vi "StateShooter.vi"(0 "Master State In":T1(ring)) -> ()   [LabVIEW 2023]
doc: "This VI performs all of the calculations and decisions related to the swerve drive."
uses:
  <vilib>/Rock Robotics/WPI/DriverStation/WPI_DriverStationAllianceInfo.ctl
  52ab7f25-ced8-4b52-a2db-c1468d392cc7.vi
  GlobalDriverStationCommands.vi
  GlobalShooter.vi
  GlobalNoteHandling.vi
  GlobalPoseAndTargeting.vi
  GlobalDriverStationData.vi
  GlobalAutonomous.vi
  GlobalElevator.vi
panel:
  in  "Stage Shooter Command":dbl=0.35 format="%#_13g"
  in  "StageAngle":dbl
  in  "AMP Shooter Command":dbl=0.5 format="%#_13g"
  in  "Speaker Height":dbl=65.0 format="%#_13g"
  in  "Shooter Ratio":dbl=-0.576 format="%#_13g"
  in  "Shooter Command":dbl=0.7 format="%#_13g"
  in  "Wrist Default angle (deg)":dbl=27.0 format="%#_13g"
  in  "Shooter Firing Duration (ms)":u32=500
  in  "Trap Wrist Angle":dbl
  in  "Climbing Wrist Angle":dbl=54.0
  in  "Amp Wrist Angle":dbl=72.0
  in  "Acceptable Wrist Error (deg)":dbl=2.0
  in  "Maximum Shooter Range (in)":dbl=240.0
  in  "Acceptable Heading Error (deg)":dbl=5.0 format="%#_13g"
  in  "Shooter_Acceptable_Velocity_Speaker (RPM)":dbl=1000.0
  in  "Prespin Duration (ms)":u32=2000
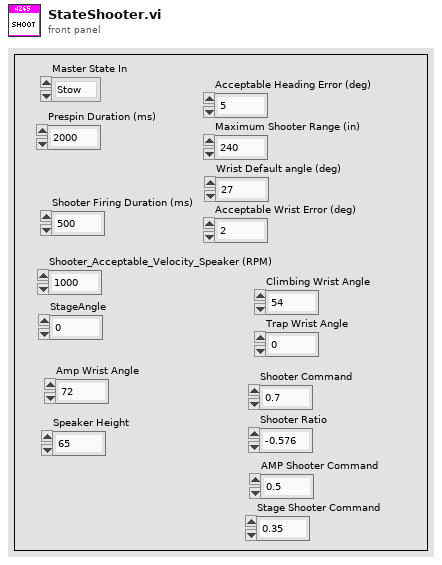
[diagram p1: front panel]
types:
  T1 = enum16{"Stow", "Speaker", "Amp", "Climbing", "Trap"}
  T2 = typedef "WPI_DriverStationAllianceInfo.ctl" = enum16{"Red", "Blue", "Invalid"}
  T3 = enum16{"Safety", "Travelling", "Positioning", "Holding"}
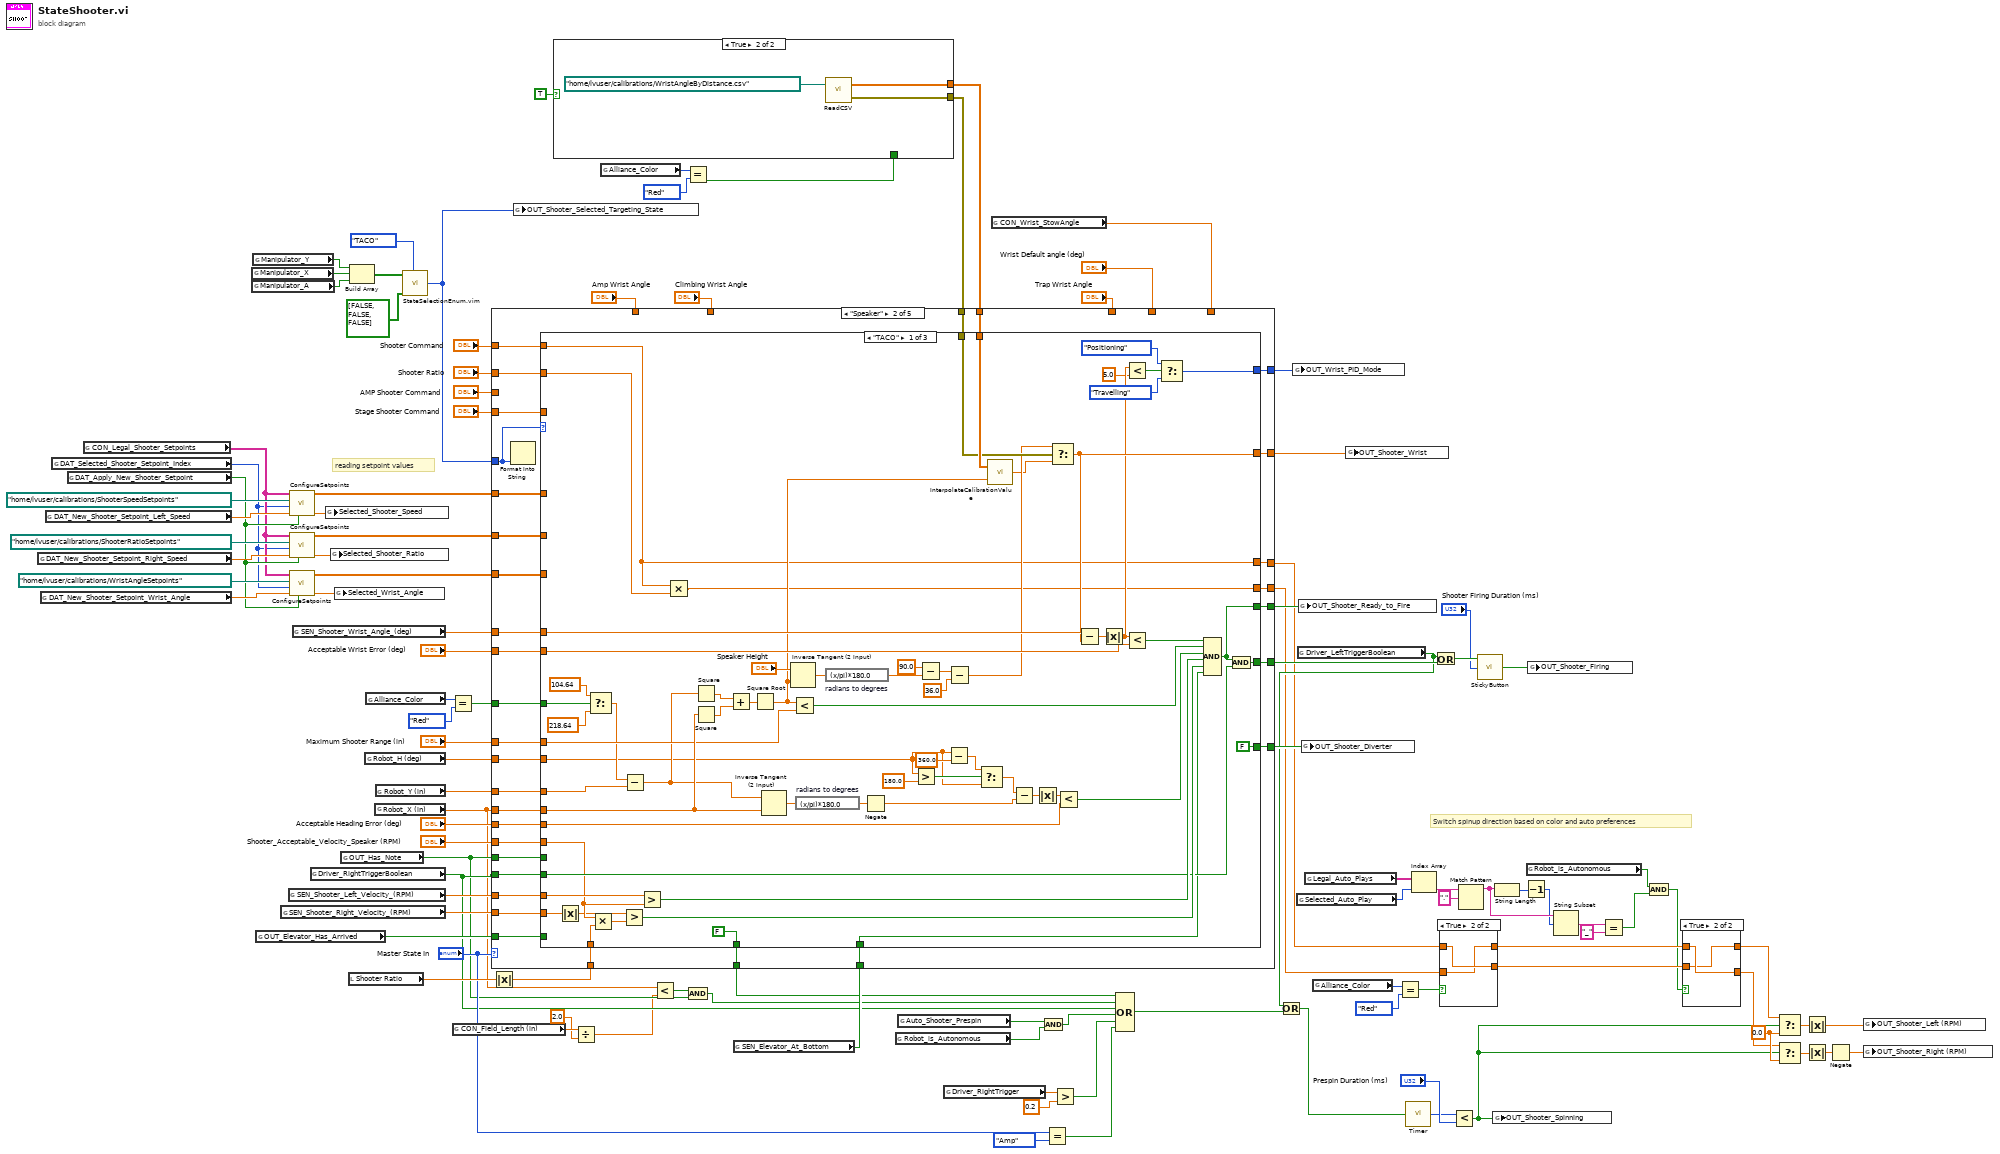
[diagram p0: block diagram]
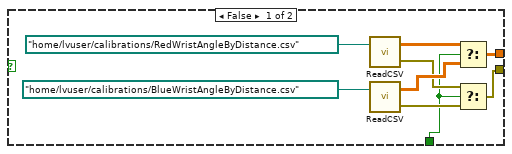
[diagram p4: hidden frame]
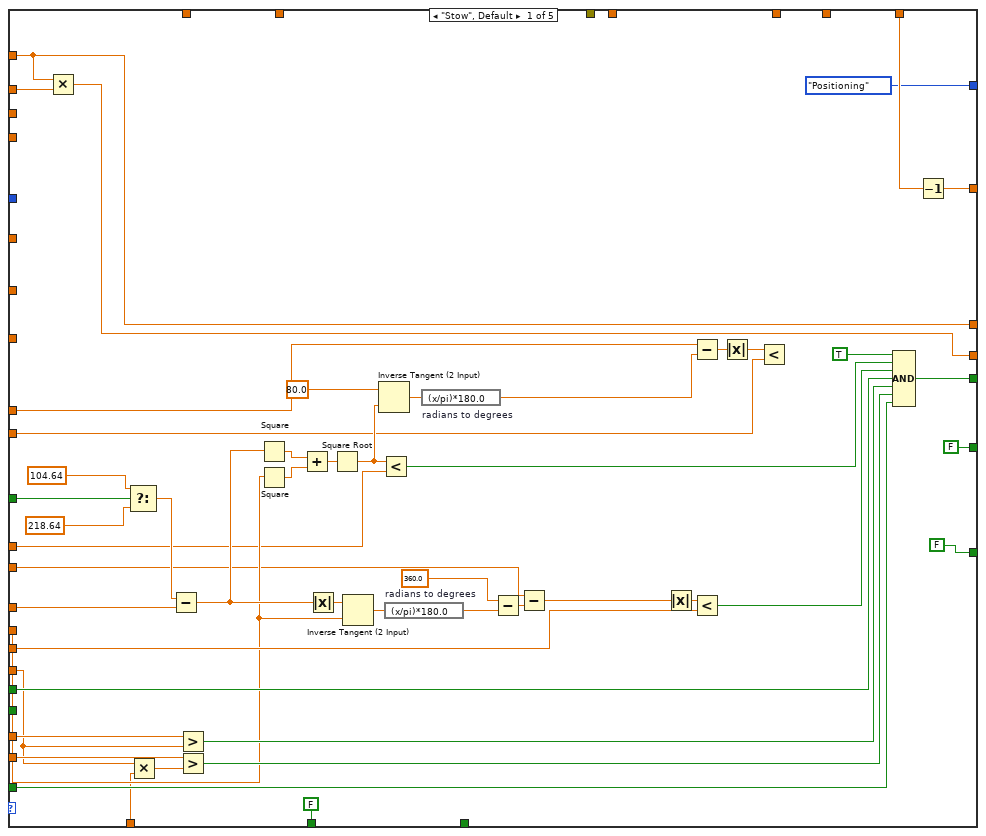
[diagram p5: hidden frame]
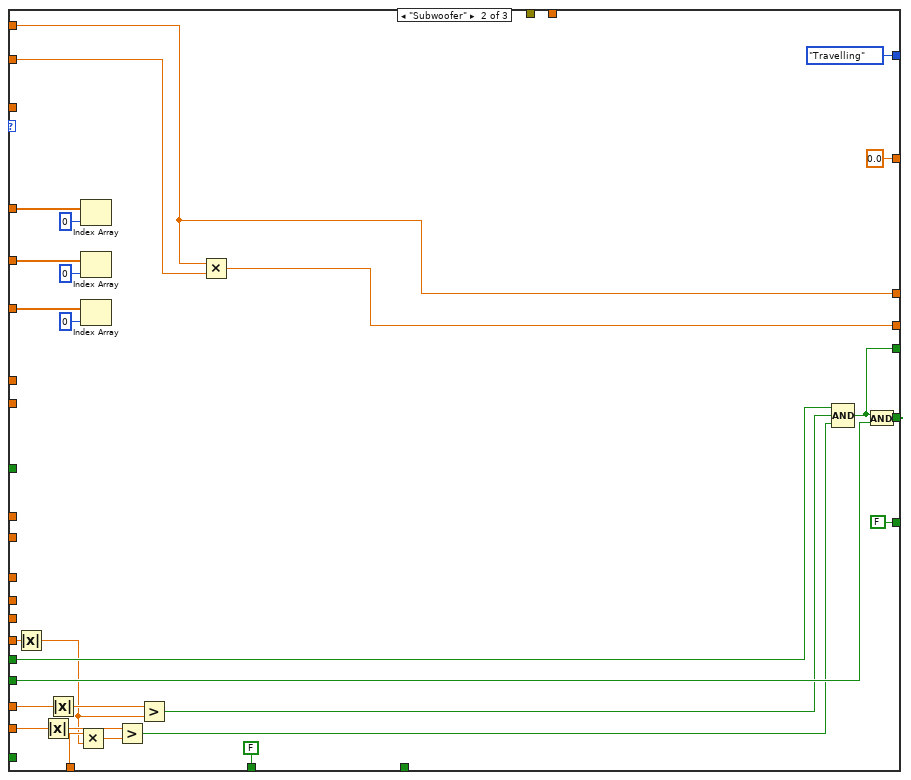
[diagram p6: hidden frame]
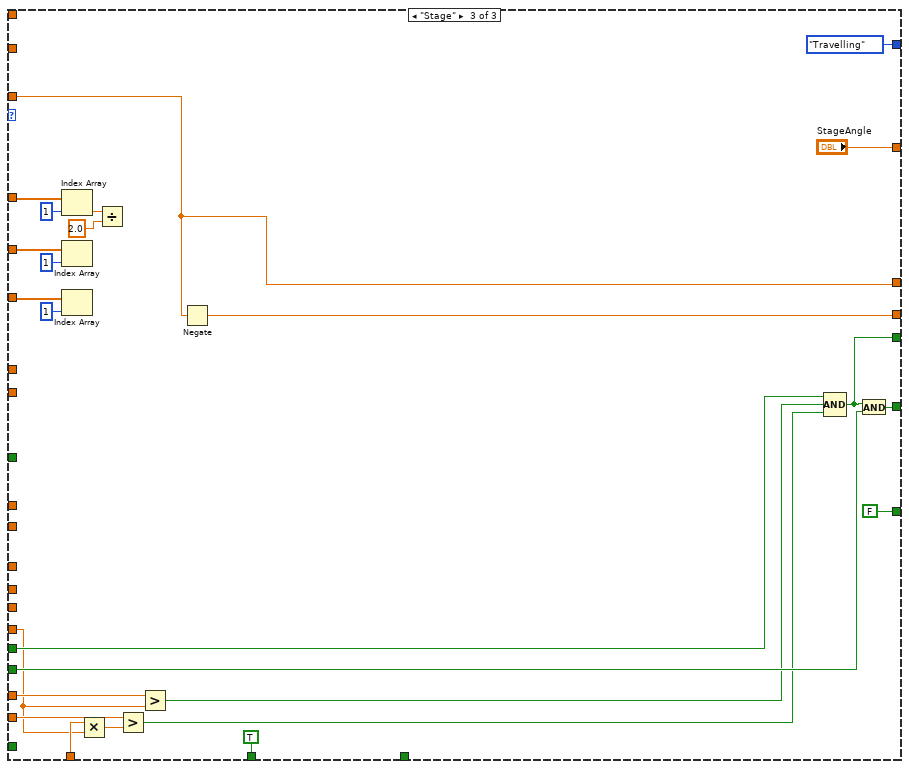
[diagram p7: hidden frame]
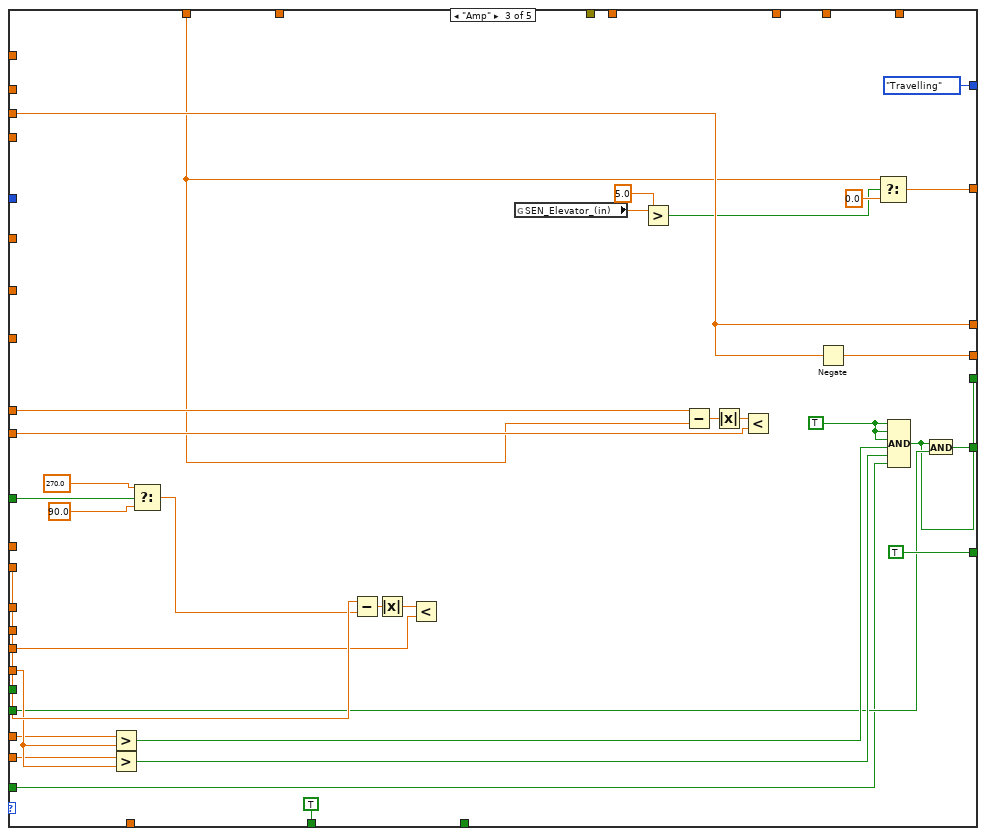
[diagram p8: hidden frame]
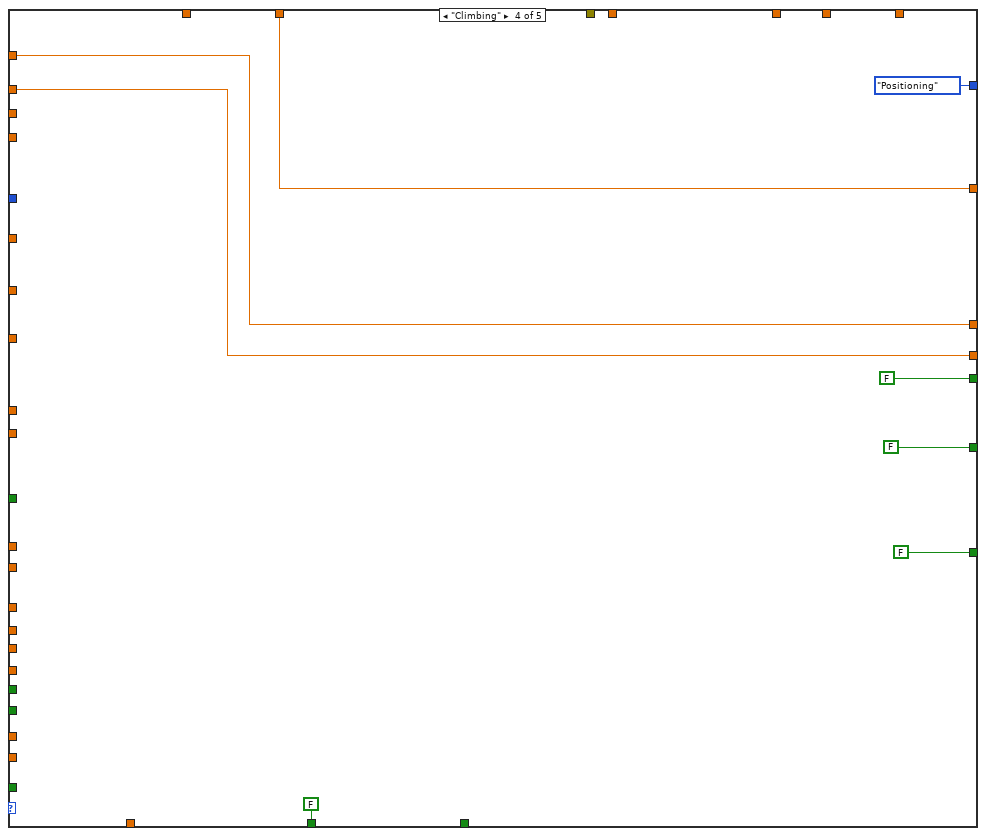
[diagram p9: hidden frame]
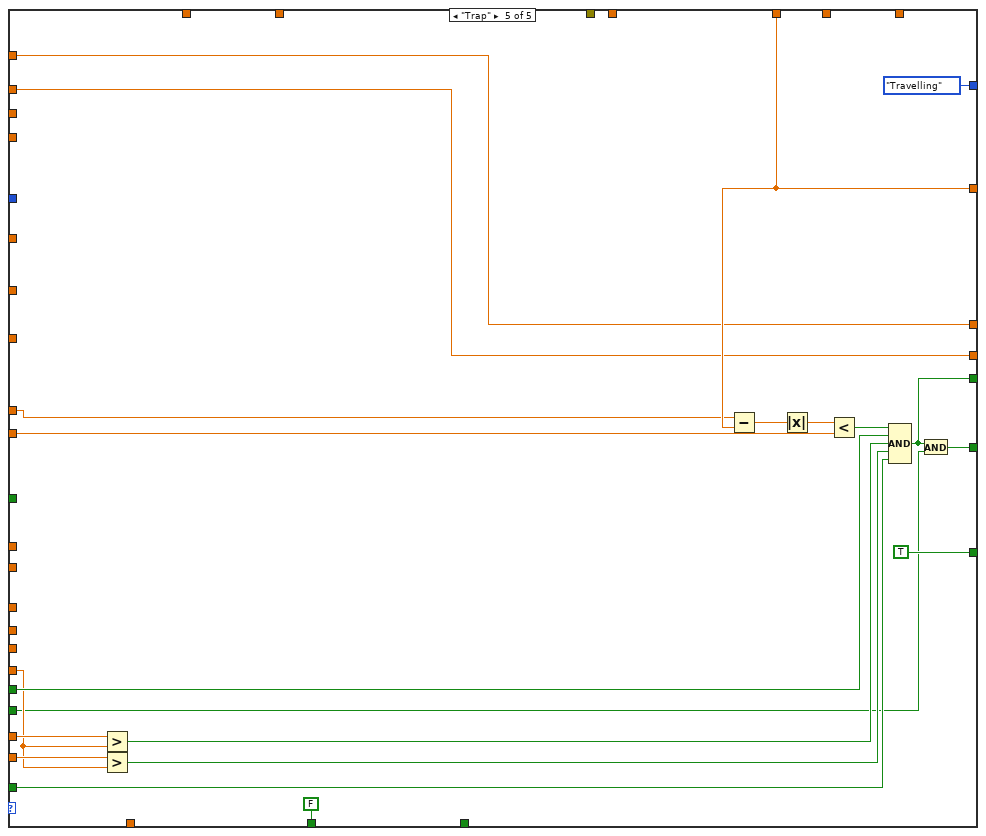
[diagram p10: hidden frame]
diagram:
  w64 = 0.0 ("f")
  # "Switch spinup direction based on color and auto preferences"
  # "reading setpoint values"
  n1 = global read "GlobalShooter.vi" "DAT_New_Shooter_Setpoint_Right_Speed"() -> (w78:dbl)
  n2 = global read "GlobalShooter.vi" "DAT_New_Shooter_Setpoint_Wrist_Angle"() -> (w75:dbl)
  n3 = global read "GlobalShooter.vi" "DAT_New_Shooter_Setpoint_Left_Speed"() -> (w79:dbl)
  n4 = global read "GlobalShooter.vi" "DAT_Selected_Shooter_Setpoint_Index"() -> (w68:i32)
  n5 = global read "GlobalShooter.vi" "DAT_Apply_New_Shooter_Setpoint"() -> (w74:bool)
  n6 = global read "GlobalShooter.vi" "CON_Legal_Shooter_Setpoints"() -> (w69:string[])
  n7 = global read "GlobalDriverStationCommands.vi" "Manipulator_X"() -> (w86:bool)
  n8 = global read "GlobalDriverStationCommands.vi" "Manipulator_A"() -> (w85:bool)
  n9 = global read "GlobalDriverStationCommands.vi" "Manipulator_Y"() -> (w87:bool)
  n10 = global read "GlobalElevator.vi" "OUT_Elevator_Has_Arrived"() -> (w57:bool)
  n11 = global read "GlobalShooter.vi" "SEN_Shooter_Right_Velocity_(RPM)"() -> (w111:dbl)
  n12 = global read "GlobalShooter.vi" "SEN_Shooter_Left_Velocity_(RPM)"() -> (w112:dbl)
  n13 = call "ConfigureSetpoints.vi"("Apply New Setpoint"=w74, "New Setpoint"=w79, "Selected Setpoint Index"=w68, "Setpoint Save Location"=path "/home/lvuser/calibrations/ShooterSpeedSetpoints", "Setpoint Names"=w69) -> ("Selected Setpoint Value"=w73:dbl, "Setpoints"=w67:dbl[])  [unwired: 5 in]
  n14 = call "ConfigureSetpoints.vi"("Apply New Setpoint"=w74, "New Setpoint"=w78, "Selected Setpoint Index"=w68, "Setpoint Save Location"=path "/home/lvuser/calibrations/ShooterRatioSetpoints", "Setpoint Names"=w69) -> ("Selected Setpoint Value"=w72:dbl, "Setpoints"=w66:dbl[])  [unwired: 5 in]
  n15 = call "ConfigureSetpoints.vi"("Apply New Setpoint"=w74, "New Setpoint"=w75, "Selected Setpoint Index"=w68, "Setpoint Save Location"=path "/home/lvuser/calibrations/WristAngleSetpoints", "Setpoint Names"=w69) -> ("Selected Setpoint Value"=w71:dbl, "Setpoints"=w65:dbl[])  [unwired: 5 in]
  n16 = global read "GlobalShooter.vi" "SEN_Shooter_Wrist_Angle_(deg)"() -> (w107:dbl)
  n17 = global read "GlobalDriverStationCommands.vi" "Driver_RightTriggerBoolean"() -> (w45:bool)
  n18 = global write "GlobalShooter.vi" "Selected_Shooter_Speed"(w73) -> ()
  n19 = global write "GlobalShooter.vi" "Selected_Shooter_Ratio"(w72) -> ()
  n20 = global write "GlobalShooter.vi" "Selected_Wrist_Angle"(w71) -> ()
  n21 = global read "GlobalNoteHandling.vi" "OUT_Has_Note"() -> (w44:bool)
  n22 = local read "Shooter Ratio"() -> (w61:dbl)
  n23 = Build Array(w87, w86, w85) -> (w88:bool[])
  n24 = global read "GlobalPoseAndTargeting.vi" "Robot_H (deg)"() -> (w106:dbl)
  n25 = global read "GlobalDriverStationData.vi" "Alliance_Color"() -> (w104:T2)
  n26 = global read "GlobalPoseAndTargeting.vi" "Robot_X (in)"() -> (w15:dbl)
  n27 = global read "GlobalPoseAndTargeting.vi" "Robot_Y (in)"() -> (w105:dbl)
  n28 = call "StateSelectionEnum.vim"("Enum Def"=enum16{"TACO", "Subwoofer", "Stage"}."TACO", "Disallowed States"=bool[] [FALSE, FALSE, FALSE], "State Triggers"=w88) -> ("Selected State"=w70:enum16{"TACO", "Subwoofer", "Stage"})  [unwired: 2 in, 1 out]
  n29 = Equal?(x=w104, y=WPI_DriverStationAllianceInfo."Red") -> (x = y?=w99:bool)
  n30 = global read "GlobalPoseAndTargeting.vi" "CON_Field_Length (in)"() -> (w14:dbl)
  n31 = Absolute Value(x=w61) -> (abs(x)=w60:dbl)
  n32 = global write "GlobalShooter.vi" "OUT_Shooter_Selected_Targeting_State"(w70) -> ()
  n33 = Divide(x=w14, y=2.0) -> (x/y=w12:dbl)
  n34 = global read "GlobalDriverStationData.vi" "Alliance_Color"() -> (w41:T2)
  n35 = Less?(x=w15, y=w12) -> (x < y?=w16:bool)
  n36 = Equal?(x=w41, y=WPI_DriverStationAllianceInfo."Red") -> (x = y?=w39:bool)
  n37 = case shown="True" TRUE {
    tunnel: [w118 w123] -> w43
    tunnel: [w114 w122] -> w10
    tunnel: w39 -> [w113 _]
    frame False {
      n38 = call "ReadCSV.vi"("File Path (.csv)"=path "/home/lvuser/calibrations/RedWristAngleByDistance.csv" ("Setpoint Save Location")) -> ("File Open Eror"=w116:errorcluster, "Data (index by row)"=w119:dbl[][])  [unwired: 1 in]
      n39 = call "ReadCSV.vi"("File Path (.csv)"=path "/home/lvuser/calibrations/BlueWristAngleByDistance.csv" ("Setpoint Save Location")) -> ("File Open Eror"=w115:errorcluster, "Data (index by row)"=w117:dbl[][])  [unwired: 1 in]
      n40 = Select(t=w119, s=w113, f=w117) -> (s? t:f=w118:dbl[][])
      n41 = Select(t=w116, s=w113, f=w115) -> (s? t:f=w114:errorcluster)
    }
    frame True {
      n42 = call "ReadCSV.vi"("File Path (.csv)"=path "/home/lvuser/calibrations/WristAngleByDistance.csv" ("Setpoint Save Location")) -> ("File Open Eror"=w122:errorcluster, "Data (index by row)"=w123:dbl[][])  [unwired: 1 in]
    }
  }
  n43 = And(x=w16, y=w44) -> (x .and. y?=w17:bool)
  n44 = global read "GlobalElevator.vi" "SEN_Elevator_At_Bottom"() -> (w53:bool)
  n45 = global read "GlobalDriverStationData.vi" "Robot_is_Autonomous"() -> (w18:bool)
  n46 = global read "GlobalAutonomous.vi" "Auto_Shooter_Prespin"() -> (w93:bool)
  n47 = global read "GlobalDriverStationCommands.vi" "Driver_RightTrigger"() -> (w83:dbl)
  n48 = global read "GlobalShooter.vi" "CON_Wrist_StowAngle"() -> (w90:dbl)
  n49 = case shown="\"Speaker\"" "Master State In" {
    tunnel: w45 -> [_ w193 w337 _ w370]
    tunnel: w112 -> [w143 w207 w344 _ w377]
    tunnel: w111 -> [w144 w206 w343 _ w378]
    tunnel: [FALSE w192 w338 FALSE w371] -> w109
    tunnel: w44 -> [w147 w197 _ _ w379]
    tunnel: "Shooter_Acceptable_Velocity_Speaker (RPM)" -> [w130 w205 w345 _ w376]
    tunnel: [w125 w190 w332 w364 w383] -> w59
    tunnel: w107 -> [w135 w194 w352 _ w382]
    tunnel: w106 -> [w139 w204 w351 _ _]
    tunnel: w105 -> [w140 w203 _ _ _]
    tunnel: w15 -> [w141 w202 _ _ _]
    tunnel: "Acceptable Heading Error (deg)" -> [w142 w201 w350 _ _]
    tunnel: "Maximum Shooter Range (in)" -> [w138 w200 _ _ _]
    tunnel: "Acceptable Wrist Error (deg)" -> [w136 w199 w346 _ w384]
    tunnel: w99 -> [w137 w198 w347 _ _]
    tunnel: "Amp Wrist Angle" -> [_ _ w330 _ _]
    tunnel: "Climbing Wrist Angle" -> [_ _ _ w364 _]
    tunnel: "Trap Wrist Angle" -> [_ _ _ _ w383]
    tunnel: w57 -> [w145 w196 w329 _ w373]
    tunnel: [FALSE w195 TRUE FALSE TRUE] -> w94
    tunnel: [w146 w191 w336 FALSE w369] -> w92
    tunnel: "Wrist Default angle (deg)" -> [_ _ _ _ _]
    tunnel: w90 -> [w174 _ _ _ _]
    tunnel: w70 -> [_ w189 _ _ _]
    tunnel: w67 -> [_ w188 _ _ _]
    tunnel: w66 -> [_ w187 _ _ _]
    tunnel: w65 -> [_ w186 _ _ _]
    tunnel: [w133 w182 w335 w360 w368] -> w35
    tunnel: "Shooter Command" -> [w133 w184 _ w360 w368]
    tunnel: [w132 w185 w334 w359 w367] -> w34
    tunnel: "Shooter Ratio" -> [w134 w183 _ w359 w367]
    tunnel: w60 -> [w131 w181 _ _ _]
    tunnel: "AMP Shooter Command" -> [_ _ w335 _ _]
    tunnel: w53 -> [_ w180 _ _ _]
    tunnel: w43 -> [_ w179 _ _ _]
    tunnel: w10 -> [_ w178 _ _ _]
    tunnel: "Stage Shooter Command" -> [_ w177 _ _ _]
    tunnel: [T3."Positioning" ("OUT_Wrist_PID_Mode") w176 T3."Travelling" ("OUT_Wrist_PID_Mode") T3."Positioning" ("OUT_Wrist_PID_Mode") T3."Travelling" ("OUT_Wrist_PID_Mode")] -> w38
    tunnel: [FALSE w175 TRUE FALSE FALSE] -> w11
    frame "Stow", Default {
      n50 = Multiply(x=w133, y=w134) -> (x*y=w132:dbl)
      n51 = Select(t=104.64 ("Robot_Y (in)"), s=w137, f=218.64 ("Robot_Y (in)")) -> (s? t:f=w149:dbl)
      n52 = Multiply(x=w130, y=w131) -> (x*y=w129:dbl)
      n53 = Subtract(x=w149, y=w140) -> (x-y=w157:dbl)
      n54 = Greater?(x=w143, y=w130) -> (0:w171:bool)
      n55 = Greater?(x=w144, y=w129) -> (0:w170:bool)
      n56 = Square(x=w157) -> (x^2=w159:dbl)
      n57 = Square(x=w141) -> (x^2=w160:dbl)
      n58 = Add(x=w159, y=w160) -> (x+y=w161:dbl)
      n59 = Absolute Value(x=w157) -> (abs(x)=w164:dbl)
      n60 = Square Root(x=w161) -> (sqrt(x)=w154:dbl)
      n61 = Inverse Tangent (2 Input)(1:w141, 2:w164) -> (0:w165:dbl)
      n62 = Inverse Tangent (2 Input)(1:w154, 2:80.0) -> (0:w156:dbl)
      n63 = Less?(x=w154, y=w138) -> (x < y?=w158:bool)
      n64 = expression code="(x/pi)*180.0" "radians to degrees"(w165) -> (w166:dbl)
      n65 = expression code="(x/pi)*180.0" "radians to degrees"(w156) -> (w148:dbl)
      n66 = Subtract(x=360.0, y=w166) -> (x-y=w167:dbl)
      n67 = Subtract(x=w139, y=w167) -> (x-y=w168:dbl)
      n68 = Absolute Value(x=w168) -> (abs(x)=w169:dbl)
      n69 = Subtract(x=w135, y=w148) -> (x-y=w152:dbl)
      n70 = Less?(x=w169, y=w142) -> (x < y?=w162:bool)
      n71 = Absolute Value(x=w152) -> (abs(x)=w153:dbl)
      n72 = Less?(x=w153, y=w136) -> ()  [unwired: 1 out]
      n73 = Compound Arithmetic op=AND(TRUE ("value"), w158, w162, w147, w171, w170, w145) -> (w146:bool)
      n74 = Decrement(x=w174) -> (x-1=w125:dbl)
    }
    frame "Speaker" {
      n75 = Format Into String(w189) -> ()  [unwired: 3 in, 2 out]
      n76 = case shown="\"TACO\"" w189 {
        tunnel: w207 -> [w271 w283 w312]
        tunnel: w206 -> [w240 w282 w311]
        tunnel: w205 -> [w241 w284 w304]
        tunnel: w204 -> [w220 _ _]
        tunnel: w203 -> [w257 _ _]
        tunnel: w202 -> [w256 _ _]
        tunnel: w201 -> [w255 _ _]
        tunnel: w200 -> [w254 _ _]
        tunnel: w199 -> [w253 _ _]
        tunnel: w198 -> [w211 _ _]
        tunnel: w197 -> [_ w294 w305]
        tunnel: w196 -> [_ _ _]
        tunnel: [FALSE FALSE FALSE] -> w195
        tunnel: w194 -> [w248 _ _]
        tunnel: w193 -> [w247 w296 w308]
        tunnel: [w246 w297 w309] -> w192
        tunnel: [w245 w295 w303] -> w191
        tunnel: [w221 0.0 ("Forward Position Wheel 4") "StageAngle"] -> w190
        tunnel: w188 -> [_ w290 w318]
        tunnel: w187 -> [_ w289 w317]
        tunnel: w186 -> [_ w288 w316]
        tunnel: [w210 w279 w301] -> w182
        tunnel: [w209 w287 w315] -> w185
        tunnel: w184 -> [w210 w279 _]
        tunnel: w183 -> [w244 w278 _]
        tunnel: w181 -> [w243 w285 w313]
        tunnel: w180 -> [w234 _ _]
        tunnel: w179 -> [w226 _ _]
        tunnel: w178 -> [w224 _ _]
        tunnel: w177 -> [_ _ w301]
        tunnel: [w214 T3."Travelling" ("OUT_Wrist_PID_Mode") T3."Travelling" ("OUT_Wrist_PID_Mode")] -> w176
        tunnel: [FALSE FALSE TRUE] -> w175
        frame "TACO" {
          n77 = Absolute Value(x=w240) -> (abs(x)=w233:dbl)
          n78 = Select(t=104.64 ("Robot_Y (in)"), s=w211, f=218.64 ("Robot_Y (in)")) -> (s? t:f=w250:dbl)
          n79 = Multiply(x=w241, y=w243) -> (x*y=w242:dbl)
          n80 = Greater?(x=w233, y=w242) -> (0:w269:bool)
          n81 = Subtract(x=w250, y=w257) -> (x-y=w232:dbl)
          n82 = Greater?(x=w271, y=w241) -> (0:w270:bool)
          n83 = Multiply(x=w210, y=w244) -> (x*y=w209:dbl)
          n84 = Square(x=w232) -> (x^2=w262:dbl)
          n85 = Square(x=w256) -> (x^2=w263:dbl)
          n86 = Add(x=w262, y=w263) -> (x+y=w264:dbl)
          n87 = Square Root(x=w264) -> (sqrt(x)=w225:dbl)
          n88 = Inverse Tangent (2 Input)(1:w256, 2:w232) -> (0:w266:dbl)
          n89 = Inverse Tangent (2 Input)(1:w225, 2:"Speaker Height") -> (0:w260:dbl)
          n90 = Less?(x=w225, y=w254) -> (x < y?=w261:bool)
          n91 = expression code="(x/pi)*180.0" "radians to degrees"(w266) -> (w231:dbl)
          n92 = expression code="(x/pi)*180.0" "radians to degrees"(w260) -> (w239:dbl)
          n93 = Negate(x=w231) -> (-x=w218:dbl)
          n94 = Greater?(x=w220, y=180.0) -> (0:w229:bool)
          n95 = Subtract(x=90.0, y=w239) -> (x-y=w237:dbl)
          n96 = Subtract(x=w220, y=360.0) -> (x-y=w227:dbl)
          n97 = Subtract(x=w237, y=36.0) -> (x-y=w223:dbl)
          n98 = Select(t=w227, s=w229, f=w220) -> (s? t:f=w219:dbl)
          n99 = call "InterpolateCalibrationValue.vi"("Input"=w225, "Calibration Data"=w226) -> ("Interpolated Output"=w222:dbl)
          n100 = Subtract(x=w219, y=w218) -> (x-y=w267:dbl)
          n101 = Absolute Value(x=w267) -> (abs(x)=w268:dbl)
          n102 = Select(t=w223, s=w224, f=w222) -> (s? t:f=w221:dbl)
          n103 = Less?(x=w268, y=w255) -> (x < y?=w265:bool)
          n104 = Subtract(x=w248, y=w221) -> (x-y=w258:dbl)
          n105 = Absolute Value(x=w258) -> (abs(x)=w217:dbl)
          n106 = Less?(x=w217, y=5.0) -> (x < y?=w215:bool)
          n107 = Less?(x=w217, y=w253) -> (x < y?=w235:bool)
          n108 = Select(t=T3."Positioning" ("OUT_Wrist_PID_Mode"), s=w215, f=T3."Travelling" ("OUT_Wrist_PID_Mode")) -> (s? t:f=w214:T3)
          n109 = Compound Arithmetic op=AND(w235, w261, w265, w270, w269, w234) -> (w245:bool)
          n110 = And(x=w245, y=w247) -> (x .and. y?=w246:bool)
        }
        frame "Subwoofer" {
          n111 = Absolute Value(x=w284) -> (abs(x)=w274:dbl)
          n112 = Absolute Value(x=w282) -> (abs(x)=w276:dbl)
          n113 = Absolute Value(x=w283) -> (abs(x)=w277:dbl)
          n114 = Multiply(x=w285, y=w274) -> (x*y=w286:dbl)
          n115 = Index Array(array=w290, index=0) -> ()  [unwired: 1 out]
          n116 = Index Array(array=w289, index=0) -> ()  [unwired: 1 out]
          n117 = Index Array(array=w288, index=0) -> ()  [unwired: 1 out]
          n118 = Greater?(x=w276, y=w286) -> (0:w280:bool)
          n119 = Greater?(x=w277, y=w274) -> (0:w281:bool)
          n120 = Multiply(x=w279, y=w278) -> (x*y=w287:dbl)
          n121 = Compound Arithmetic op=AND(w294, w281, w280) -> (w295:bool)
          n122 = And(x=w295, y=w296) -> (x .and. y?=w297:bool)
        }
        frame "Stage" {
          n123 = Index Array(array=w318, index=1) -> (element=w319:dbl)
          n124 = Index Array(array=w317, index=1) -> ()  [unwired: 1 out]
          n125 = Index Array(array=w316, index=1) -> ()  [unwired: 1 out]
          n126 = Multiply(x=w313, y=w304) -> (x*y=w314:dbl)
          n127 = Divide(x=w319, y=2.0) -> ()  [unwired: 1 out]
          n128 = Greater?(x=w311, y=w314) -> (0:w307:bool)
          n129 = Greater?(x=w312, y=w304) -> (0:w306:bool)
          n130 = Negate(x=w301) -> (-x=w315:dbl)
          n131 = Compound Arithmetic op=AND(w305, w306, w307) -> (w303:bool)
          n132 = And(x=w303, y=w308) -> (x .and. y?=w309:bool)
        }
      }
    }
    frame "Amp" {
      w333 = TRUE ("value")
      n133 = Greater?(x=w344, y=w345) -> (0:w341:bool)
      n134 = Greater?(x=w343, y=w345) -> (0:w342:bool)
      n135 = Select(t=270.0 ("Robot_Y (in)"), s=w347, f=90.0 ("Robot_Y (in)")) -> (s? t:f=w339:dbl)
      n136 = Subtract(x=w351, y=w339) -> (x-y=w354:dbl)
      n137 = Absolute Value(x=w354) -> (abs(x)=w353:dbl)
      n138 = Less?(x=w353, y=w350) -> ()  [unwired: 1 out]
      n139 = global read "GlobalElevator.vi" "SEN_Elevator_(in)"() -> (w328:dbl)
      n140 = Greater?(x=w328, y=5.0) -> (0:w326:bool)
      n141 = Subtract(x=w352, y=w330) -> (x-y=w356:dbl)
      n142 = Absolute Value(x=w356) -> (abs(x)=w355:dbl)
      n143 = Less?(x=w355, y=w346) -> ()  [unwired: 1 out]
      n144 = Negate(x=w335) -> (-x=w334:dbl)
      n145 = Select(t=w330, s=w326, f=0.0) -> (s? t:f=w332:dbl)
      n146 = Compound Arithmetic op=AND(w333, w333, w333, w341, w342, w329) -> (w336:bool)
      n147 = And(x=w336, y=w337) -> (x .and. y?=w338:bool)
    }
    frame "Climbing" {
    }
    frame "Trap" {
      n148 = Greater?(x=w377, y=w376) -> (0:w375:bool)
      n149 = Greater?(x=w378, y=w376) -> (0:w374:bool)
      n150 = Subtract(x=w382, y=w383) -> (x-y=w381:dbl)
      n151 = Absolute Value(x=w381) -> (abs(x)=w385:dbl)
      n152 = Less?(x=w385, y=w384) -> (x < y?=w380:bool)
      n153 = Compound Arithmetic op=AND(w380, w379, w375, w374, w373) -> (w369:bool)
      n154 = And(x=w369, y=w370) -> (x .and. y?=w371:bool)
    }
  }
  n155 = And(x=w93, y=w18) -> (x .and. y?=w19:bool)
  n156 = Equal?(x="Master State In", y=T1."Amp") -> (x = y?=w54:bool)
  n157 = Greater?(x=w83, y=0.2) -> (0:w81:bool)
  n158 = Compound Arithmetic op=OR(w11, w17, w45, w19, w81, w54) -> (w48:bool)
  n159 = global write "GlobalShooter.vi" "OUT_Wrist_PID_Mode"(w38) -> ()
  n160 = global read "GlobalDriverStationData.vi" "Selected_Auto_Play"() -> (w27:u16)
  n161 = global read "GlobalDriverStationCommands.vi" "Driver_LeftTriggerBoolean"() -> (w49:bool)
  n162 = Or(x=w49, y=w48) -> (x .or. y?=w47:bool)
  n163 = global write "GlobalShooter.vi" "OUT_Shooter_Ready_to_Fire"(w92) -> ()
  n164 = global write "GlobalShooter.vi" "OUT_Shooter_Diverter"(w94) -> ()
  n165 = global read "GlobalAutonomous.vi" "Legal_Auto_Plays"() -> (w28:string[])
  n166 = global read "GlobalDriverStationData.vi" "Alliance_Color"() -> (w31:T2)
  n167 = global write "GlobalShooter.vi" "OUT_Shooter_Wrist"(w59) -> ()
  n168 = Equal?(x=w31, y=WPI_DriverStationAllianceInfo."Red") -> (x = y?=w29:bool)
  n169 = call "Timer.vi"("Reset Timer"=w47) -> ("Time (ms)"=w95:u32)
  n170 = Index Array(array=w28, index=w27) -> (element=w8:string)
  n171 = Or(x=w49, y=w109) -> (x .or. y?=w52:bool)
  n172 = case shown="True" w29 {
    tunnel: w35 -> [w387 w389]
    tunnel: [w387 w388] -> w37
    tunnel: w34 -> [w386 w388]
    tunnel: [w386 w389] -> w36
    frame False {
    }
    frame True {
    }
  }
  n173 = Less?(x=w95, y="Prespin Duration (ms)") -> (x < y?=w46:bool)
  n174 = Match Pattern(string=w8, regular expression=".") -> (before substring=w6:string)  [unwired: 1 in, 3 out]
  n175 = call "StickyButton.vi"("Time threshold (ms)"="Shooter Firing Duration (ms)", "Button Input"=w52) -> ("Sticky Button"=w50:bool)  [unwired: 1 in]
  n176 = global write "GlobalShooter.vi" "OUT_Shooter_Spinning"(w46) -> ()
  n177 = String Length(string=w6) -> (length=w5:i32)
  n178 = Decrement(x=w5) -> (x-1=w4:i32)
  n179 = global read "GlobalDriverStationData.vi" "Robot_is_Autonomous"() -> (w25:bool)
  n180 = global write "GlobalShooter.vi" "OUT_Shooter_Firing"(w50) -> ()
  n181 = String Subset(string=w6, offset (0)=w4) -> (substring=w3:string)  [unwired: 1 in]
  n182 = Equal?(x=w3, y="_") -> (x = y?=w1:bool)
  n183 = And(x=w25, y=w1) -> (x .and. y?=w26:bool)
  n184 = case shown="True" w26 {
    tunnel: w37 -> [w391 w393]
    tunnel: [w391 w392] -> w33
    tunnel: w36 -> [w390 w392]
    tunnel: [w390 w393] -> w32
    frame False {
    }
    frame True {
    }
  }
  n185 = Select(t=w33, s=w46, f=w64) -> (s? t:f=w24:dbl)
  n186 = Select(t=w32, s=w46, f=w64) -> (s? t:f=w22:dbl)
  n187 = Absolute Value(x=w24) -> (abs(x)=w23:dbl)
  n188 = Absolute Value(x=w22) -> (abs(x)=w21:dbl)
  n189 = Negate(x=w21) -> (-x=w20:dbl)
  n190 = global write "GlobalShooter.vi" "OUT_Shooter_Left (RPM)"(w23) -> ()
  n191 = global write "GlobalShooter.vi" "OUT_Shooter_Right (RPM)"(w20) -> ()
